vi "gvboolesch_ECD.vi"() -> ()   [LabVIEW 2017]
panel:
  in  "global stop":bool
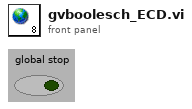
[diagram p1: front panel]
diagram:
